vi "SortAccordingToZ.vi"(8 "error in (no error)":errorcluster, 10 "Parameters":T2={"number of planes"=4, "z step"=1.9999999999999998e-05, "pixel dwell time"=1.0000000000000001e-11, "z frequency"=10.0, "number of pixels"=100, "smooth points"=10, "smooth line"=10, "Sine\nSawtooth"=FALSE, "PointSorting"=0, "Sort Points"=FALSE, "X-pixels"=256.0, "Y-lines"=256.0, "pixelstoµm"=256.0, "zoom"=1.0, "Time offset"=1.0000000000000001e-11} {"zoom" min=0.5 step=0.1; "Y-lines" min=1 step=1; "X-pixels" min=1 step=1; "PointSorting" items=["No Difference", "Every Second Point", "Down / Up"]; "smooth line" min=1; "smooth points" min=1; "number of pixels" min=1; "z frequency" format="%_4g"; "number of planes" min=1}, 11 "XYZ Point coordinates (pixels)":dbl[][](array[numeric])) -> (0 "error out":errorcluster, 2 "DutyCluster":T1 {"Iteration" items=["first iteration", "second iteration"]}, 3 "XYZ Point coordinates updated (pixels)":dbl[][](array[numeric]))   [LabVIEW 2010]
uses:
  TypeDefs/ParameterCluster.ctl
  TypeDefs/DutyCluster.ctl
panel:
  out "min index":dbl
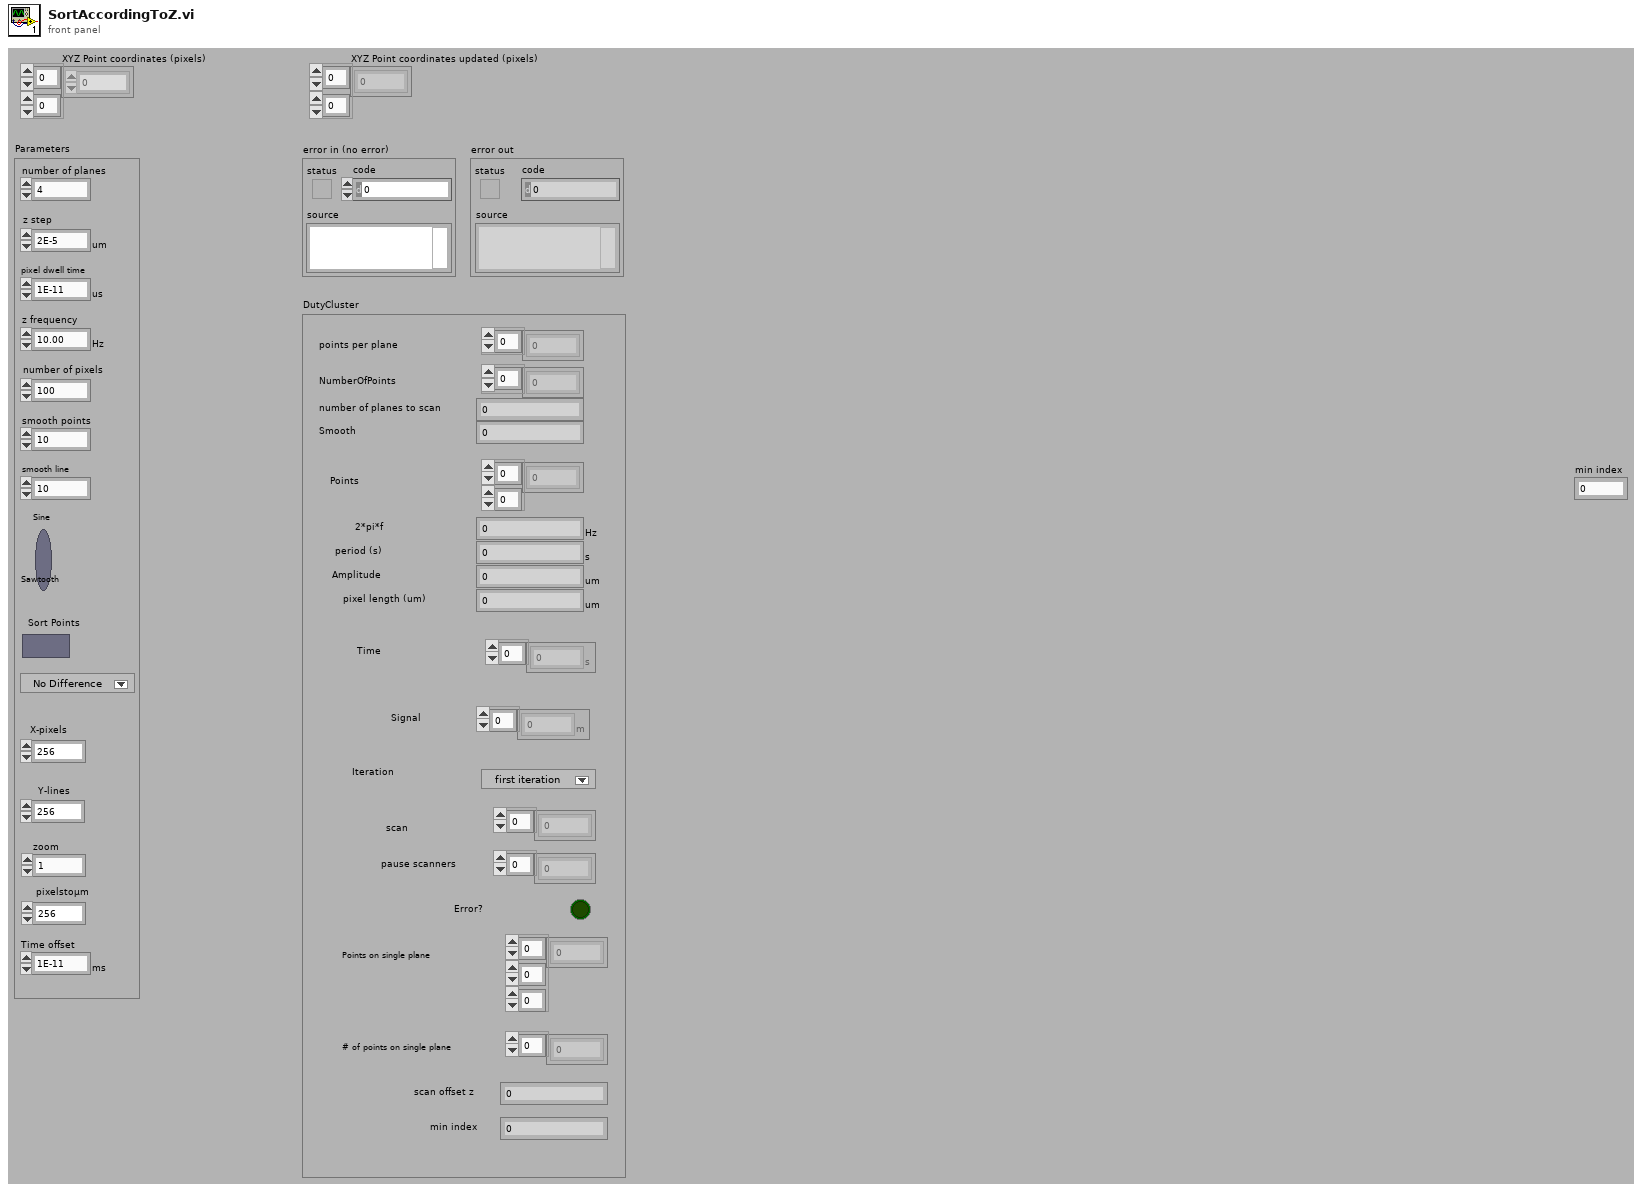
[diagram p1: front panel]
types:
  T1 = typedef "DutyCluster.ctl" = cluster{"points per plane":i32[], "NumberOfPoints":i32[], "number of planes to scan":i32, "Smooth":i32, "Points":dbl[][], "2*pi*f":dbl[unit], "period (s)":dbl[unit], "Amplitude":dbl[unit], "pixel length (um)":dbl[unit], "Time":dbl[unit][], "Signal":dbl[unit][], "Iteration":u16, "scan":i32[], "pause scanners":i32[], "Error?":bool, "Points on single plane":dbl[][][], "# of points on single plane":i32[], "scan offset z":i32, "min index":i32}
  T2 = typedef "ParameterCluster.ctl" = cluster{"number of planes":i32, "z step":dbl[unit], "pixel dwell time":dbl[unit], "z frequency":dbl[unit], "number of pixels":i32, "smooth points":i32, "smooth line":i32, "Sine\nSawtooth":bool, "PointSorting":u16, "Sort Points":bool, "X-pixels":sgl, "Y-lines":sgl, "pixelstoµm":dbl, "zoom":dbl, "Time offset":dbl[unit]}
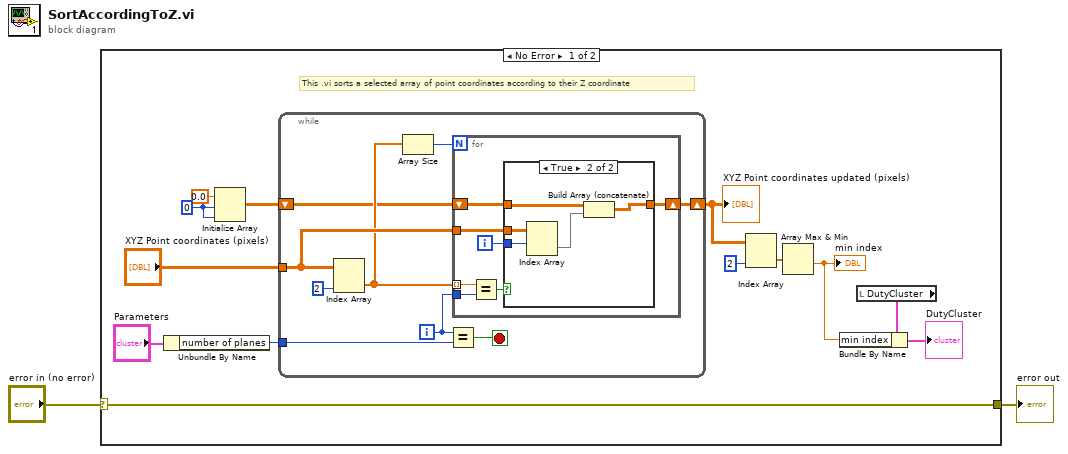
[diagram p0: block diagram]
diagram:
  n1 = case shown="No Error" "error in (no error)" {
    selector: "error in (no error)" -> [w11 w38]
    tunnel: [w11 w38] -> w1
    frame No Error {
      w13 = 0 ("dimension size")
      # "This .vi sorts a selected array of point coordinates according to their Z coordinate"
      n2 = Unbundle By Name("Parameters") -> ("number of planes"=w9:i32)
      n3 = Initialize Array(0.0 ("element"), w13, w13) -> (w14:dbl[][])
      n4 = while {
        tunnel: "XYZ Point coordinates (pixels)" -> [w23]
        shift-right: [w17] -> w6
        shift-left: w14 -> [w18]
        tunnel: w9 -> [w16]
        i -> [w20]
        stop <- w21 stop-if-true
        n5 = Index Array(array=w23, index (col)=2 ("disabled index (col)")) -> (element=w22:dbl[])  [unwired: 1 in]
        n6 = Array Size(array=w22) -> (size(s)=w19:i32)
        n7 = Equal?(x=w20, y=w16) -> (x = y?=w21:bool)
        n8 = for {
          N: w19 -> [_]
          tunnel: w22 -> [w31] mode=indexing
          tunnel: w23 -> [w29]
          shift-right: [w28] -> w17
          shift-left: w18 -> [w27]
          tunnel: w20 -> [w26]
          i -> [w25]
          n9 = Equal?(x=w31, y=w26) -> (x = y?=w30:bool)
          n10 = case shown="True" w30 {
            tunnel: w29 -> [_ w37]
            tunnel: w25 -> [_ w33]
            tunnel: [w32 w36] -> w28
            tunnel: w27 -> [w32 w35]
            frame False {
            }
            frame True {
              n11 = Index Array(array=w37, index (row)=w33) -> (element=w34:dbl[])  [unwired: 1 in]
              n12 = Build Array (concatenate)(w35, w34) -> (w36:dbl[][])
            }
          }
        }
      }
      "XYZ Point coordinates updated (pixels)" <- w6
      n13 = Index Array(array=w6, index (col)=2 ("disabled index (col)")) -> (element=w7:dbl[])  [unwired: 1 in]
      n14 = Array Max & Min(array=w7) -> (min value=w5:dbl)  [unwired: 3 out]
      "min index" <- w5
      n15 = local read "DutyCluster"() -> (w4:T1)
      n16 = Bundle By Name(cluster=w4, "min index"=w5) -> (→"DutyCluster":T1)
    }
    frame Error {
    }
  }
  "error out" <- w1
